vi "transform.vi"(6 "offset":refnum<class "SpaceVector.lvclass">, 7 "zoom":dbl=1.0, 8 "error in (no error)":errorcluster, 9 "x angle (psi)":dbl[unit], 10 "z angle (phi)":dbl[unit], 11 "TrajectoryAK101022Resonance in":refnum<class "TrajectoryAK101022Resonance.lvclass">) -> (0 "error out":errorcluster, 3 "TrajectoryAK101022Resonance out":refnum<class "TrajectoryAK101022Resonance.lvclass">)   [LabVIEW 2010, in "TrajectoryAK101022Resonance.lvclass"]
uses:
  TrajectoryAK101022Resonance.lvclass
  common/classes/SpaceVector/SpaceVector/SpaceVector.lvclass
  TrajectoryMG100122GenericFPGA/TrajectoryMG100122GenericFPGA/TrajectoryMG100122GenericFPGA.lvclass
  TrajectoryAK101022Resonance.lvclass/TrajectoryAK101022Resonance.ctl
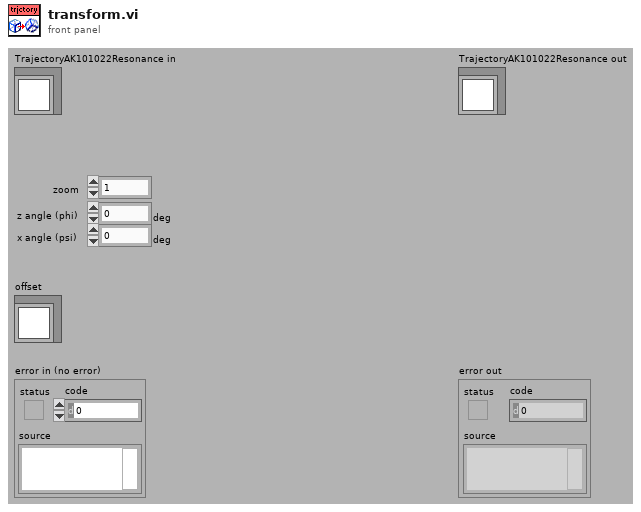
[diagram p1: front panel]
types:
  T1 = typedef "scan_specification_cluster.ctl" = cluster{"x amplitude":u16, "x resolution (pixels)":u16, "x offset fly-forward (iterations)":u16, "x offset fly-back (iterations)":u16, "y resolution (nr. of lines)":u16, "y step size":u16, "iterations per pixel":u16, "number of frames":i32, "y offset (pixels)":u16, "number of y-brake lines  (before y-fly-back)":u16, "number y-brake lines (after y-fly-back)":u16, "y-fly-back step size":u16, "number of y-fly-back steps":u16}
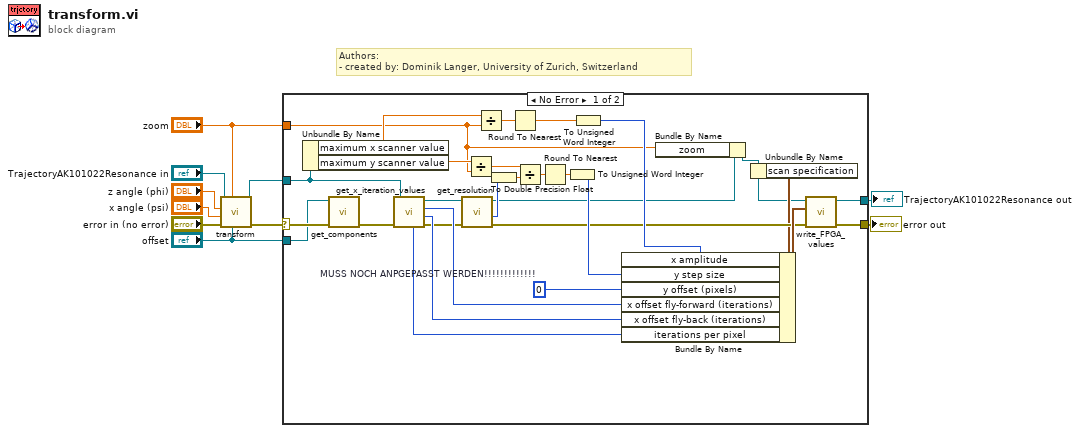
[diagram p0: block diagram]
diagram:
  # "Authors: \n- created by: Dominik Langer, University of Zurich, Switzerland"
  n1 = call-parent "transform.vi"("SpaceVector.lvclass"="offset", "zoom"="zoom", "error in (no error)"="error in (no error)", "x angle (psi)"="x angle (psi)", "z angle (phi)"="z angle (phi)", "TrajectoryMG100122GenericFPGA in"="TrajectoryAK101022Resonance in") -> ("error out"=w6:errorcluster, "TrajectoryMG100122GenericFPGA out"=w5:refnum<class "TrajectoryAK101022Resonance.lvclass">)  [unwired: 4 in]
  n2 = case shown="No Error" w6 {
    selector: w6 -> [w33 w40]
    tunnel: w5 -> [w28 w41]
    tunnel: "zoom" -> [w15 _]
    tunnel: "offset" -> [w31 _]
    tunnel: [w39 w40] -> w2
    tunnel: [w38 w41] -> w1
    frame No Error {
      w16 = u16 0  # MUSS NOCH ANPGEPASST WERDEN!!!!!!!!!!!!!
      n3 = Unbundle By Name(w28) -> ("maximum x scanner value"=w26:dbl, "maximum y scanner value"=w25:dbl)
      n4 = call "get_components.vi"("error in (no error)"=w33, "SpaceVector in"=w31) -> ("error out"=w32:errorcluster)  [unwired: 4 in, 5 out]
      n5 = call-dynamic "get_x_iteration_values.vi"("error in (no error)"=w32, "TrajectoryAK101022Resonance in"=w28) -> ("error out"=w23:errorcluster, "fly-back offset [iterations]"=w35:u16, "fly-forward offset [iterations]"=w37:u16, "TrajectoryAK101022Resonance out"=w24:refnum<class "TrajectoryAK101022Resonance.lvclass">, "iterations per pixel"=w34:u16)  [unwired: 4 in, 1 out]
      n6 = call-dynamic "get_resolution.vi"("error in (no error)"=w23, "TrajectoryAK101022Resonance in"=w24) -> ("error out"=w13:errorcluster, "y resolution"=w21:i32, "TrajectoryAK101022Resonance out"=w14:refnum<class "TrajectoryAK101022Resonance.lvclass">)  [unwired: 6 in, 1 out]
      n7 = Divide(x=w25, y=w15) -> (x/y=w22:dbl)
      n8 = Divide(x=w26, y=w15) -> (x/y=w27:dbl)
      n9 = To Double Precision Float(number=w21) -> (double precision float=w20:dbl)
      n10 = Round To Nearest(number=w27) -> (nearest integer value=w30:dbl)
      n11 = Divide(x=w22, y=w20) -> (x/y=w18:dbl)
      n12 = Round To Nearest(number=w18) -> (nearest integer value=w19:dbl)
      n13 = To Unsigned Word Integer(number=w19) -> (unsigned 16bit integer=w17:u16)
      n14 = To Unsigned Word Integer(number=w30) -> (unsigned 16bit integer=w29:u16)
      n15 = Bundle By Name(cluster=w14, "zoom"=w15) -> (w11:refnum<class "TrajectoryAK101022Resonance.lvclass">)
      n16 = Unbundle By Name(w11) -> ("scan specification"=w12:T1)
      n17 = Bundle By Name(cluster=w12, "x amplitude"=w29, "y step size"=w17, "y offset (pixels)"=w16, "x offset fly-forward (iterations)"=w37, "x offset fly-back (iterations)"=w35, "iterations per pixel"=w34) -> (w36:T1)
      n18 = call-dynamic "write_FPGA_values.vi"("error in (no error)"=w13, "scan specification"=w36, "TrajectoryAK101022Resonance in"=w11) -> ("error out"=w39:errorcluster, "TrajectoryAK101022Resonance out"=w38:refnum<class "TrajectoryAK101022Resonance.lvclass">)  [unwired: 7 in]
    }
    frame Error {
    }
  }
  "error out" <- w2
  "TrajectoryAK101022Resonance out" <- w1
